vi "Realization of Gates using NOR Gates.vi"() -> ()   [LabVIEW 2021]
panel:
  in  "B":bool
  out "Output of OR":bool
  in  "A":bool
  out "Output of the AND":bool
  in  "B":bool
  in  "A":bool
  out "Output of NOT":bool
  in  "A":bool
  # "NOT GATE"
  # "OR GATE"
  # "AND GATE"
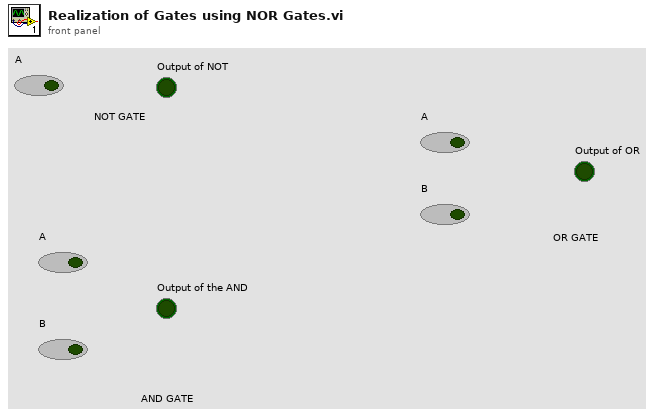
[diagram p1: front panel]
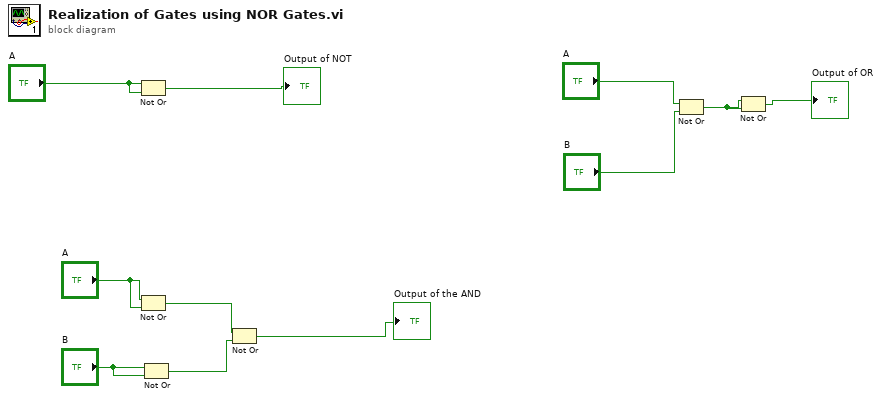
[diagram p0: block diagram]
diagram:
  n1 = Not Or(1:"A", 2:"A") -> (0:→"Output of NOT":bool)
  n2 = Not Or(1:"A", 2:"A") -> (0:w6:bool)
  n3 = Not Or(1:"B", 2:"B") -> (0:w7:bool)
  n4 = Not Or(1:w7, 2:w6) -> (0:→"Output of the AND":bool)
  n5 = Not Or(1:"B", 2:"A") -> (0:w2:bool)
  n6 = Not Or(1:w2, 2:w2) -> (0:→"Output of OR":bool)
